vi "XNET Write (Frame LIN).vi"(0 "session in":refnum<k21>, 5 "data":T1[](array[typedef]) {"event ID" format="%x"; "payload" format="%x"; "timestamp" format="%<%.7X\n%x>T"; "type" items=["LIN Data"=64, "LIN Bus Error"=65, "LIN No Response"=66, "Delay"=224, "Log Trigger"=225, "Start Trigger"=226]; "identifier" format="%x"}, 9 "timeout (10)":dbl=10.0 format="%.2g", 11 "error in (no error)":errorcluster) -> (4 "session out":refnum<k21>, 15 "error out":errorcluster)   [LabVIEW 2018]
doc: "Writes data to a session as an array of LIN frames. The session must use a LIN interface and a mode of Frame Output Stream, Frame Output Queued, or Frame Output Single-Point."
uses:
  XNET Frame LIN.ctl
  XNET Frame Type LIN.ctl
  nixlvapi.dll
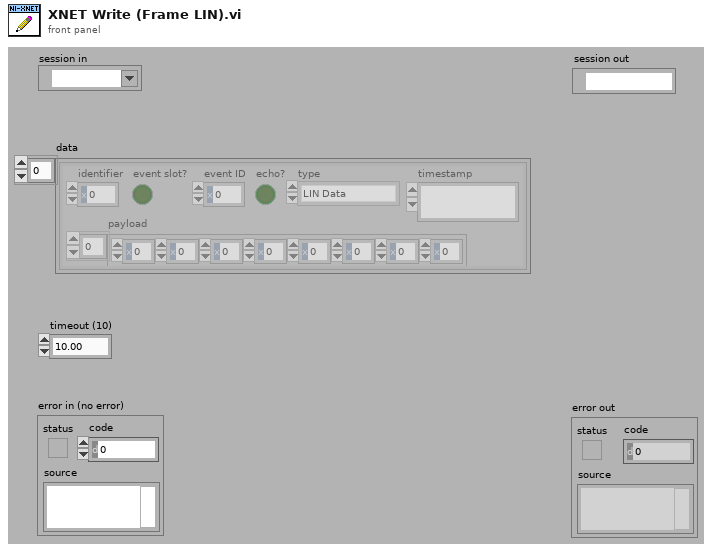
[diagram p1: front panel]
types:
  T1 = typedef "XNET Frame LIN.ctl" = cluster{"timestamp":timestamp, "payload":u8[], "identifier":u32, "type":T2, "event ID":u8, "event slot?":bool, "echo?":bool}
  T2 = typedef "XNET Frame Type LIN.ctl" = u8
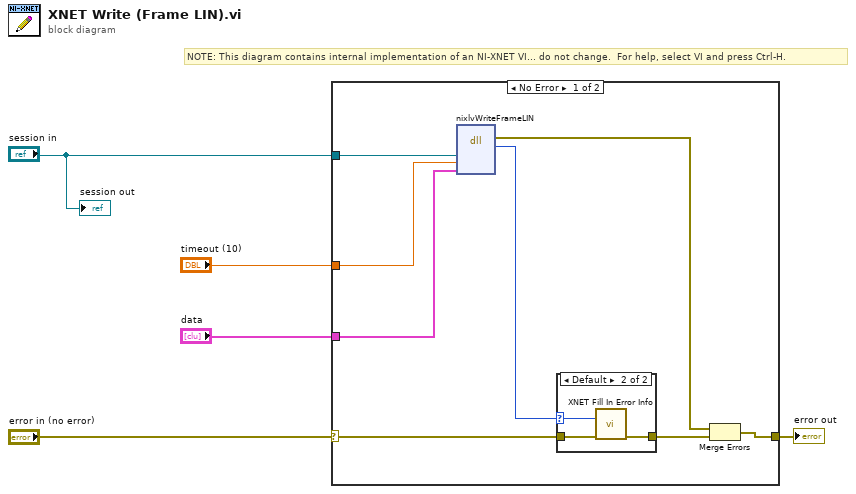
[diagram p0: block diagram]
diagram:
  # "NOTE: This diagram contains internal implementation of an NI-XNET VI... do not change.  For help, select VI and press Ctrl-H."
  n1 = case shown="No Error" "error in (no error)" {
    selector: "error in (no error)" -> [w12 w18]
    tunnel: "session in" -> [w13 _]
    tunnel: [w8 w18] -> w5
    tunnel: "timeout (10)" -> [w10 _]
    tunnel: "data" -> [w9 _]
    frame No Error {
      n2 = dll-call lib="nixlvapi.*" fn="nixlvWriteFrameLIN"("SessionRef"=w13, "Timeout"=w10, "Data"=w9) -> (error out=w7:errorcluster, "return type"=w11:i32)  [unwired: 5 in, 2 out]
      n3 = case shown="Default" w11 {
        selector: w11 -> [_ w15]
        tunnel: w12 -> [w14 w16]
        tunnel: [w14 w17] -> w6
        frame 0 {
        }
        frame Default {
          n4 = call "XNET Fill In Error Info.vi"("status code"=w15, "error in"=w16) -> ("error out"=w17:errorcluster)  [unwired: 13 out]
        }
      }
      n5 = Merge Errors(w7, w6) -> (w8:errorcluster)
    }
    frame Error {
    }
  }
  "error out" <- w5
  "session out" <- "session in"
